vi "Insert CVT Data.vi"(7 "Group":string, 8 "error in":errorcluster, 9 "Data":variant, 10 "tag":string, 11 "Controller in":refnum<class "Controller.lvclass">) -> (0 "error out":errorcluster, 3 "Controller out":refnum<class "Controller.lvclass">)   [LabVIEW 2014]
uses:
  Controller.lvclass
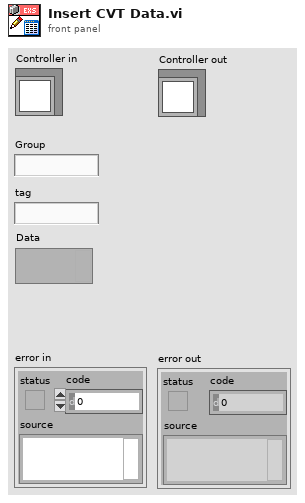
[diagram p1: front panel]
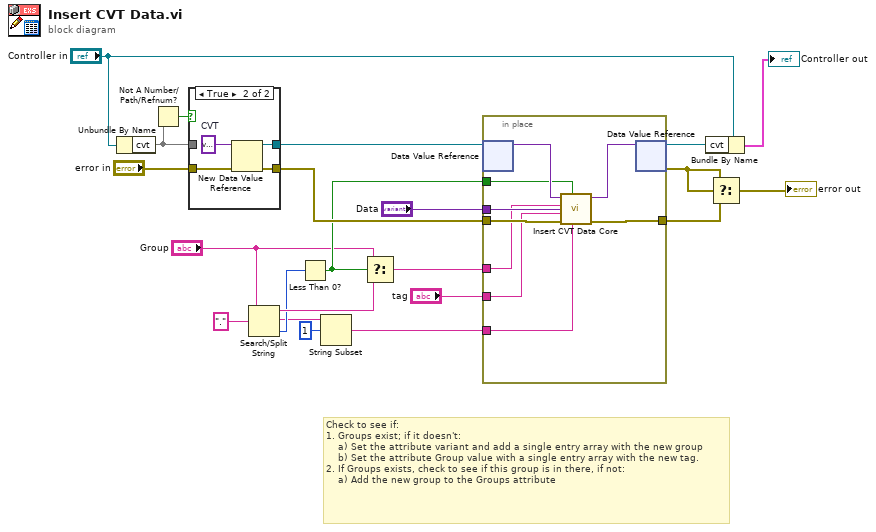
[diagram p0: block diagram]
diagram:
  # "Check to see if:\n1. Groups exist; if it doesn't:\n    a) Set the attribute variant and add a single entry array with the new group\n    b) Set the attribute Group value with a single entry array with the new tag.\n2. If Groups exists, check to see if this group is in there, if not:\n    a) Add the new group to the Groups attribute"
  n1 = Unbundle By Name("Controller in") -> ("cvt"=w13)
  n2 = Not A Number/Path/Refnum?(number/path/refnum=w13) -> (NaN/Path/Refnum?=w14:bool)
  n3 = case shown="True" w14 {
    tunnel: w13 -> [w24 _]
    tunnel: [w24 w27] -> w12
    tunnel: "error in" -> [w23 w26]
    tunnel: [w23 w25] -> w10
    frame False {
    }
    frame True {
      w28 = variant  # CVT
      n4 = New Data Value Reference(data value=w28, error in=w26) -> (data value reference=w27:refnum<data-value>, error out=w25:errorcluster)
    }
  }
  n5 = Search/Split String(string="Group", search string/char (-)="." ("regular expression")) -> (substring before match=w7:string, match + rest of string=w3:string, offset of match=w6:i32)  [unwired: 1 in]
  n6 = Less Than 0?(x=w6) -> (x < 0?=w8:bool)
  n7 = String Subset(string=w3, offset (0)=1) -> (substring=w1:string)  [unwired: 1 in]
  n8 = Select(t="Group", s=w8, f=w7) -> (s? t:f=w9:string)
  n9 = in-place {
    in-place-border: w9 -> [w30]
    in-place-border: "tag" -> [w33]
    in-place-border: "Data" -> [w36]
    in-place-border: w10 -> [w34]
    in-place-border: [w32] -> w16
    in-place-border: w8 -> [w31]
    in-place-border: w1 -> [w29]
    n10 = in-place-dvr #1(w12) -> (w37:variant)  [unwired: 1 out]
    n11 = call "Insert CVT Data Core.vi"("Data"=w36, "Nested Group"=w29, "Nested?"=w31, "error in (no error)"=w34, "tag"=w33, "Group"=w30, "CVT In"=w37) -> ("error out"=w32:errorcluster, "CVT Out"=w35:variant)  [unwired: 2 in]
    n12 = in-place-dvr #1(w35) -> (w19:refnum<data-value>, w17:errorcluster)
  }
  n13 = Bundle By Name(cluster="Controller in", "cvt"=w19) -> (→"Controller out":cluster{})
  n14 = Select(t=w17, s=w17, f=w16) -> (s? t:f=→"error out":errorcluster)
